vi "AddToEnd.vi"(3 "Array in":dbl[](array[numeric]), 5 "Data Entry":dbl) -> (0 "Array out":dbl[](array[numeric]))   [LabVIEW 2017]
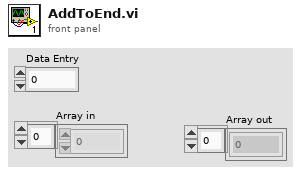
[diagram p1: front panel]
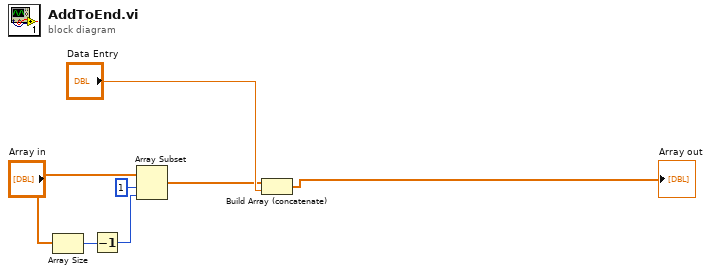
[diagram p0: block diagram]
diagram:
  n1 = Array Size(array="Array in") -> (size(s)=w1:i32)
  n2 = Decrement(x=w1) -> (x-1=w4:i32)
  n3 = Array Subset(array="Array in", index=1, length=w4) -> (w5:dbl[])
  n4 = Build Array (concatenate)(w5, "Data Entry") -> (→"Array out":dbl[])
